vi "Actor Core.vi"(8 "error in":errorcluster, 11 "uService Template in":refnum<class "Father of all uServices.lvclass">) -> (0 "error out":errorcluster, 3 "Actor out":refnum<class "Actor.lvclass">)   [LabVIEW 2026, in "TALOS.lvlib" / "Father of all uServices.lvlib" / "Father of all uServices.lvclass"]
doc: "(<B>Filename</B>: Actor Framework.lvlib:Actor.lvclass:Actor Core.vi)\n\nReceives messages to the actor, reacts to them, and initiates any error handling that may shut the actor down.\n\nDescendant classes may override this VI to append parallel tasks for the actor to complete while it handles messages. Overrides use the Call Parent Class Method node."
uses:
  Father of all uServices.lvclass
  C:/LabVIEW Code/TALOS/builds/Actor Framework PPL/Actor Framework.lvlibp/1abvi3w/vi.lib/ActorFramework/Actor/Actor.lvclass
  C:/LabVIEW Code/TALOS/talos/Ancestor/Ancestor/Ancestor.lvclass
  builds/Actor Framework PPL/Actor Framework.lvlibp/1abvi3w/vi.lib/ActorFramework/Actor/Actor.lvclass
  Father of all uServices.lvclass/Father of all uServices.ctl
  Ancestor/Ancestor/Ancestor.lvclass/Ancestor.ctl
  Father of all uServices Messages/Event Handler Msg/Event Handler Msg.lvclass/Event Handler Msg.ctl
  builds/Actor Framework PPL/Actor Framework.lvlibp/1abvi3w/vi.lib/ActorFramework/Message Enqueuer/Message Priority.ctl
  Ancestor/Ancestor Messages/Process EH Error Msg/Process EH Error Msg.lvclass/Process EH Error Msg.ctl
  19c69bdc-969d-4c15-9573-1bad74759838.vi
  Ancestor/Ancestor/Read ID.vi
  Support VIs/Generate Error.vi
  FGV/Error Memory/Get Error Description.vi
  Support VIs/Get PC name.vi
  Support VIs/Get Class Name.vi
  <vilib>/Utility/error.llb/Clear Errors.vi
  FGV/Error Memory/Error Memory Core.vi
  <vilib>/AdvancedString/Delimited String to 1D String Array.vi
  <vilib>/AdvancedString/Delimited String to 1D String Array (string).vi
  Support VIs/Circus Root Path.vi
  FGV/Error Memory/Error Crt Lvl checker.vi
  FGV/Error Memory/Error Memory Core.vi/40c8088d-b597-4017-91af-faa98e00292e.vi
  FGV/Error Memory/Error Memory Core.vi/d4a3ab98-063c-4e44-b43d-fbdcfe6c2be2.vi
  Support VIs/Global Memory.vi
  <vilib>/Utility/LVClass/Get LV Class Name.vi
  Support VIs/Is in Packed Library.vi
  Support VIs/TALOS Root path.vi
  Support VIs/Read CSV worksheet.vi
  Support VIs/Global Constants.vi
  <vilib>/Utility/error.llb/General Error Handler.vi
  Support VIs/Error Log.vi
  builds/Actor Framework PPL/Actor Framework.lvlibp/1abvi3w/vi.lib/ActorFramework/Message Enqueuer/Enqueue.vi
  Ancestor/Ancestor/Ancestor.lvclass
  <vilib>/Comparison/Equal/Equal Functor/Equal Functor.lvclass
  Father of all uServices Messages/Event Handler Msg/Event Handler Msg.lvclass
  Father of all uServices Messages/Pat 3.0 Msg/Pat 3.0 Msg.lvclass
  Ancestor/Ancestor Messages/Process EH Error Msg/Process EH Error Msg.lvclass
  builds/Actor Framework PPL/Actor Framework.lvlibp/1abvi3w/vi.lib/ActorFramework/Message Enqueuer/Message Enqueuer.lvclass
  TALOS.lvlib
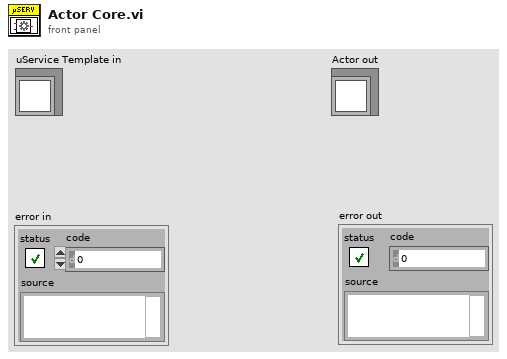
[diagram p1: front panel]
types:
  T1 = cluster{"Stop Helper Loop":refnum<user-event>, "Msg Received Event":refnum<user-event>, "Event":refnum<user-event>}
  T2 = typedef "Actor Framework.lvlibp/Message Enqueuer.lvclass/Message Priority.ctl" = enum16{"Low", "Normal", "High"}
  T3 = typedef "TALOS.lvlib/Father of all uServices.lvlib/Father of all uServices.lvclass/Msg to uServ Selector.ctl" = enum16{"Test string"}
  T4 = typedef "TALOS.lvlib/Father of all uServices.lvlib/Father of all uServices.lvclass/Event Handler Items.ctl" = enum16{"Button Pressed", "Message", "Ready to launch?", "Safe Mode", "Start RUN", "Stop RUN"}
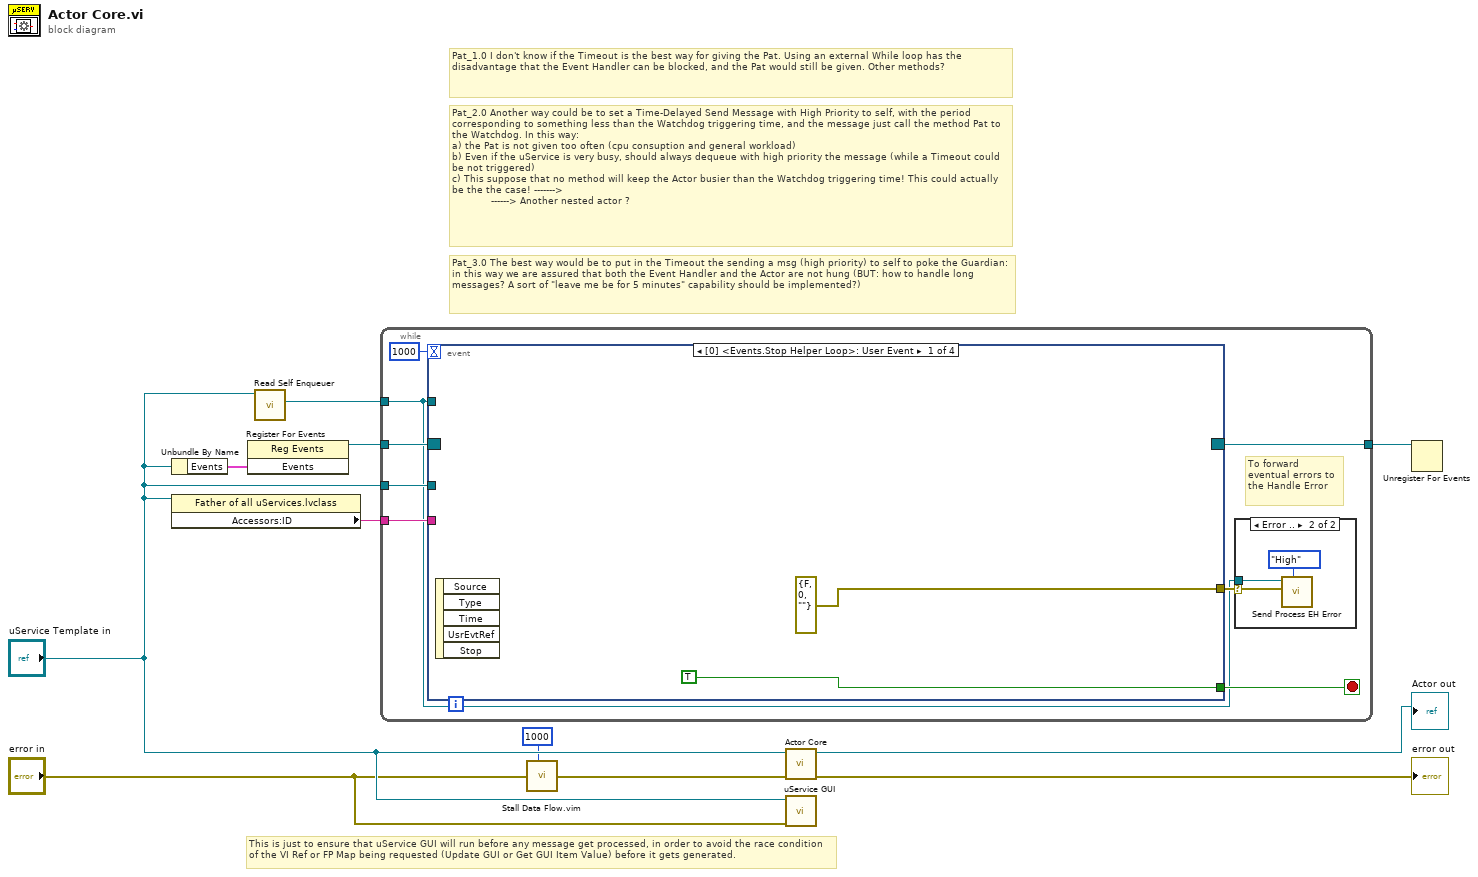
[diagram p0: block diagram]
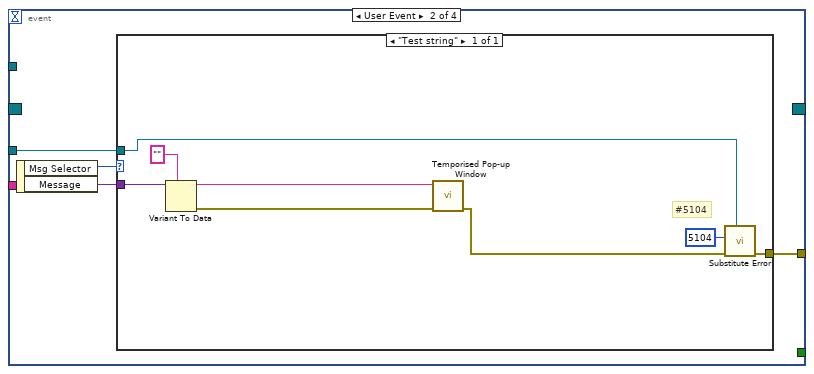
[diagram p3: hidden frame]
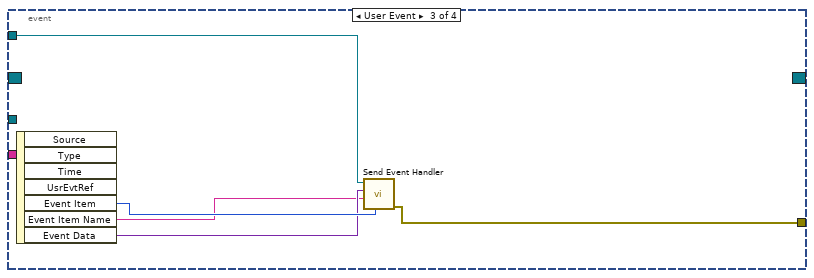
[diagram p4: hidden frame]
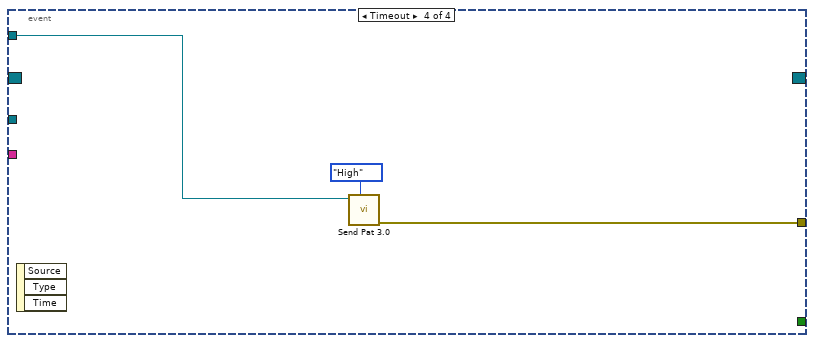
[diagram p5: hidden frame]
diagram:
  # "This is just to ensure that uService GUI will run before any message get processed, in order to avoid the race condition of the VI Ref or FP Map being requested (Update GUI or Get GUI Item Value) before it gets generated."
  # "Pat_3.0 The best way would be to put in the Timeout the sending a msg (high priority) to self to poke the Guardian: in this way we are assured that both the Event Handler and the Actor are not hung (BUT: how to handle long messages? A sort of \"leave me be for 5 minutes\" capability should be implemented?)"
  # "Pat_2.0 Another way could be to set a Time-Delayed Send Message with High Priority to self, with the period corresponding to something less than the Watchdog triggering time, and the message just call the method Pat to the Watchdog. In this way:\na) the Pat is not given too often (cpu consuption and general workload)\nb) Even if the uService is very busy, should always dequeue with high priority the message (while a Timeout could be not triggered)\nc) This suppose that no method will keep the Actor busier than the Watchdog triggering time! This could actually be the the case! ------->\n             ------> Another nested actor ?"
  # "Pat_1.0 I don't know if the Timeout is the best way for giving the Pat. Using an external While loop has the disadvantage that the Event Handler can be blocked, and the Pat would still be given. Other methods?"
  n1 = Unbundle By Name("uService Template in") -> ("Events"=w9:T1)
  n2 = property on="Property Node" class="Father of all uServices.lvclass"(reference="uService Template in") -> ("Accessors:ID"=w5:string)  [unwired: 1 in, 2 out]
  n3 = register-events(w9) -> (reference out=w8:refnum<event-registration>)  [unwired: 2 in, 1 out]
  n4 = call "Read Self Enqueuer.vi"("Actor"="uService Template in") -> ("Self Enqueuer"=w7:refnum<class "Message Enqueuer.lvclass">)  [unwired: 10 in]
  n5 = while {
    tunnel: w8 -> [w19]
    tunnel: w7 -> [w13]
    tunnel: "uService Template in" -> [w16]
    tunnel: w5 -> [w15]
    tunnel: [w12] -> w1
    stop <- w18 stop-if-true
    # "To forward eventual errors to the Handle Error"
    n6 = event shown="[0] <Events.Stop Helper Loop>: User Event" {
      selector: w19 -> [_ _ _ _]
      dyn-events: [_ _ _ _] -> w12
      timeout: 1000 -> [_ _ _ _]
      tunnel: [TRUE _ _ _] -> w18
      tunnel: w16 -> [_ w26 _ _]
      tunnel: [errorcluster {"status"=FALSE, "code"=0, "source"=""} ("error out") w25 w37 w42] -> w14
      tunnel: w15 -> [_ _ _ _]
      tunnel: w13 -> [_ _ w38 w43]
      event User Event {
        n7 = event-data() -> ()  [unwired: 1 in, 5 out]
      }
      event User Event {
        n8 = event-data() -> ("Msg Selector"=w28:T3, "Message"=w27:variant)  [unwired: 1 in]
        n9 = case shown="\"Test string\"" w28 {
          tunnel: w27 -> [w34]
          tunnel: w26 -> [w29]
          tunnel: [w36] -> w25
          frame "Test string" {
            # "#5104"
            n10 = Variant To Data(type="", Variant=w34) -> (data=w31:string, error out=w32:errorcluster)  [unwired: 1 in]
            n11 = call "Temporised Pop-up Window.vi"("error in (no error)"=w32, "Text"=w31) -> ("error out"=w30:errorcluster)  [unwired: 9 in]
            n12 = call "Substitute Error.vi"("LabVIEW Object"=w29, "error in (no error)"=w30, "Error Code"=5104) -> ("error out"=w36:errorcluster)  [unwired: 8 in]
          }
        }
      }
      event User Event {
        n13 = event-data() -> ("Event Item"=w41:T4, "Event Item Name"=w39:string, "Event Data"=w40:variant)  [unwired: 1 in, 4 out]
        n14 = call "Send Event Handler.vi"("Event type"=w41, "Item Name"=w39, "Data"=w40, "Message Enqueuer"=w38) -> ("error out"=w37:errorcluster)  [unwired: 6 in, 1 out]
      }
      event Timeout {
        n15 = event-data() -> ()  [unwired: 1 in, 3 out]
        n16 = call "Send Pat 3.0.vi"("Message Priority (Normal)"=Message_Priority."High", "Message Enqueuer"=w43) -> ("error out"=w42:errorcluster)  [unwired: 8 in, 1 out]
      }
    }
    n17 = case shown="Error .." w14 {
      selector: w14 -> [_ w22]
      tunnel: w13 -> [_ w21]
      frame No Error {
      }
      frame Error {
        n18 = call "Send Process EH Error.vi"("Message Priority (Normal)"=Message_Priority."High", "Error to process"=w22, "Message Enqueuer"=w21) -> ()  [unwired: 7 in, 2 out]
      }
    }
  }
  n19 = call "Stall Data Flow.vim"("value in"="error in", "milliseconds to wait"=u32 1000) -> ("value out"=w4:errorcluster)  [unwired: 1 out]
  n20 = call-parent "Actor Core.vi"("error in"=w4, "Actor in"="uService Template in") -> ("error out"=→"error out":errorcluster, "Actor out"=→"Actor out":refnum<class "Actor.lvclass">)  [unwired: 8 in]
  n21 = call-dynamic "uService GUI.vi"("error in (no error)"="error in", "uService Template in"="uService Template in") -> ()  [unwired: 9 in, 1 out]
  n22 = Unregister For Events(event registration refnum=w1) -> ()  [unwired: 1 in, 1 out]
